vi "Convert Number to Module.vi"(10 "input":dbl) -> (1 "Negative Module":dbl, 2 "Positive Module":dbl)   [LabVIEW 2017]
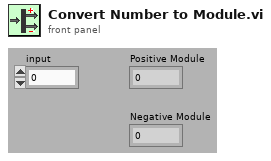
[diagram p1: front panel]
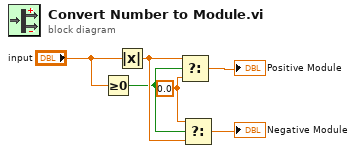
[diagram p0: block diagram]
diagram:
  w3 = 0.0 ("f")
  n1 = Greater Or Equal To 0?(x="input") -> (x >= 0?=w4:bool)
  n2 = Absolute Value(x="input") -> (abs(x)=w5:dbl)
  n3 = Select(t=w5, s=w4, f=w3) -> (s? t:f=→"Positive Module":dbl)
  n4 = Select(t=w3, s=w4, f=w5) -> (s? t:f=→"Negative Module":dbl)
